vi "Power Source Settings.vi"(8 "error in":errorcluster, 10 "Action":T1(ring), 11 "COM":refnum<visa-resource-name>="COM3") -> (0 "error out":errorcluster, 3 "read buffer":string)   [LabVIEW 2014]
uses:
  <vilib>/Instr/_visa.llb/VISA Configure Serial Port (Instr).vi
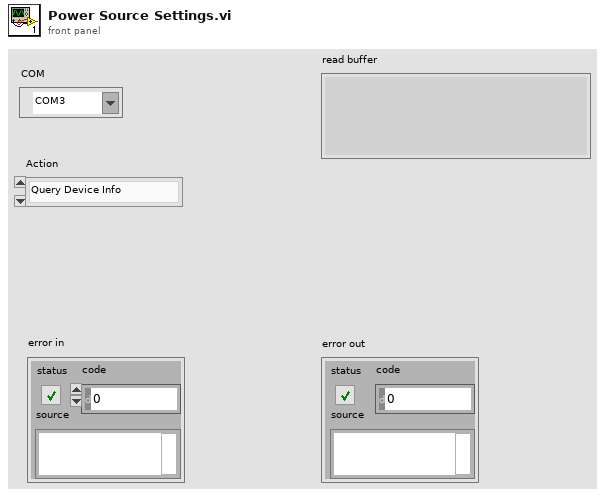
[diagram p1: front panel]
types:
  T1 = enum16{"Query Device Info", "Set Voltage", "Read Voltage", "Set Current", "Read Current", "Enable Output", "Disable Output", "Set to Remote", "Set to Local", "Get Errors", "Set Protect Voltage", "Read Protect Voltage"}
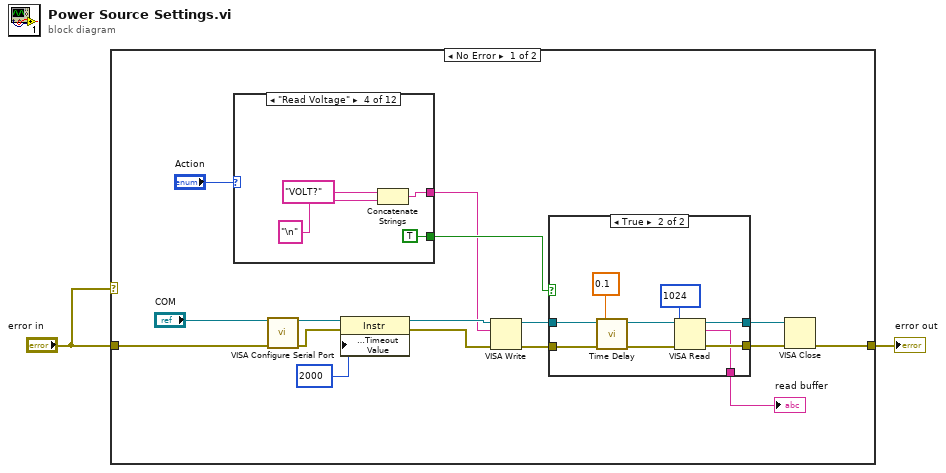
[diagram p0: block diagram]
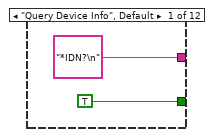
[diagram p2: hidden frame]
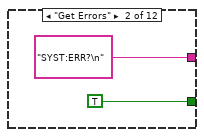
[diagram p3: hidden frame]
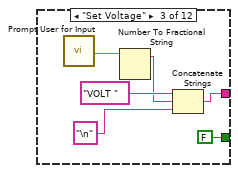
[diagram p4: hidden frame]
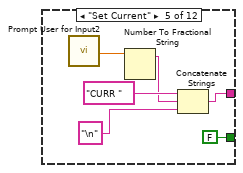
[diagram p5: hidden frame]
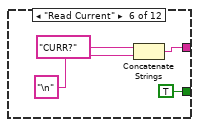
[diagram p6: hidden frame]
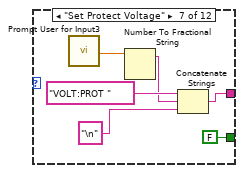
[diagram p7: hidden frame]
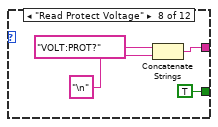
[diagram p8: hidden frame]
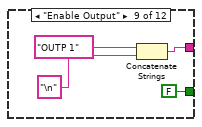
[diagram p9: hidden frame]
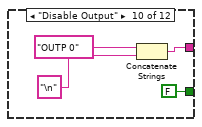
[diagram p10: hidden frame]
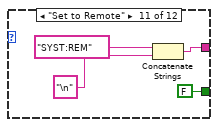
[diagram p11: hidden frame]
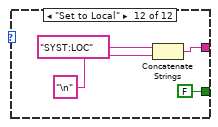
[diagram p12: hidden frame]
diagram:
  n1 = case shown="No Error" "error in" {
    tunnel: [w10 w79] -> w2
    tunnel: "error in" -> [w6 w79]
    frame No Error {
      n2 = case shown="\"Read Voltage\"" "Action" {
        tunnel: [TRUE TRUE FALSE TRUE FALSE TRUE FALSE TRUE FALSE FALSE FALSE FALSE] -> w4
        tunnel: ["*IDN?\n" ("Command") "SYST:ERR?\n" ("Command") w24 w30 w34 w40 w44 w50 w54 w58 w62 w66] -> w3
        frame "Query Device Info", Default {
        }
        frame "Get Errors" {
        }
        frame "Set Voltage" {
          n3 = call "Prompt User for Input"() -> ("电压（V)"=w27:dbl)  [unwired: 17 in, 2 out]
          n4 = Number To Fractional String(number=w27) -> (F-format string=w26:string)  [unwired: 3 in]
          n5 = Concatenate Strings("VOLT " ("Command"), w26, "\n") -> (w24:string)
        }
        frame "Read Voltage" {
          n6 = Concatenate Strings("VOLT?" ("Command"), "\n") -> (w30:string)
        }
        frame "Set Current" {
          n7 = call "Prompt User for Input2"() -> ("电流（A)"=w37:dbl)  [unwired: 17 in, 2 out]
          n8 = Number To Fractional String(number=w37) -> (F-format string=w36:string)  [unwired: 3 in]
          n9 = Concatenate Strings("CURR " ("Command"), w36, "\n") -> (w34:string)
        }
        frame "Read Current" {
          n10 = Concatenate Strings("CURR?" ("Command"), "\n") -> (w40:string)
        }
        frame "Set Protect Voltage" {
          n11 = call "Prompt User for Input3"() -> ("电压（V）"=w47:dbl)  [unwired: 17 in, 2 out]
          n12 = Number To Fractional String(number=w47) -> (F-format string=w46:string)  [unwired: 3 in]
          n13 = Concatenate Strings("VOLT:PROT " ("Command"), w46, "\n") -> (w44:string)
        }
        frame "Read Protect Voltage" {
          n14 = Concatenate Strings("VOLT:PROT?" ("Command"), "\n") -> (w50:string)
        }
        frame "Enable Output" {
          n15 = Concatenate Strings("OUTP 1" ("Command"), "\n") -> (w54:string)
        }
        frame "Disable Output" {
          n16 = Concatenate Strings("OUTP 0" ("Command"), "\n") -> (w58:string)
        }
        frame "Set to Remote" {
          n17 = Concatenate Strings("SYST:REM" ("Command"), "\n") -> (w62:string)
        }
        frame "Set to Local" {
          n18 = Concatenate Strings("SYST:LOC" ("Command"), "\n") -> (w66:string)
        }
      }
      n19 = call-poly "VISA Configure Serial Port"("VISA resource name"="COM", "error in (no error)"=w6) -> ("VISA resource name out"=w12:refnum<visa-resource-name>, "error out"=w8:errorcluster)  [unwired: 12 in]
      n20 = property class="Instr"(reference=w12, error in=w8, "General Settings:Timeout Value"=u32 2000) -> (reference out=w11:refnum<visa-resource-name>, error out=w9:errorcluster)
      n21 = VISA Write(VISA resource name=w11, write buffer=w3, error in (no error)=w9) -> (VISA resource name out=w7:refnum<visa-resource-name>, error out=w18:errorcluster)  [unwired: 1 out]
      n22 = case shown="True" w4 {
        tunnel: w18 -> [w69 w78]
        tunnel: [w69 w77] -> w17
        tunnel: [w70 w76] -> w16
        tunnel: [_ w75] -> w15
        tunnel: w7 -> [w70 w71]
        frame False {
        }
        frame True {
          n23 = call "Time Delay"("error in (no error)"=w78, "Delay Time (s)"=0.1) -> ("error out"=w73:errorcluster)  [unwired: 9 in]
          n24 = VISA Read(VISA resource name=w71, byte count=u32 1024, error in (no error)=w73) -> (VISA resource name out=w76:refnum<visa-resource-name>, read buffer=w75:string, error out=w77:errorcluster)  [unwired: 1 out]
        }
      }
      "read buffer" <- w15
      n25 = VISA Close(VISA resource name=w16, error in (no error)=w17) -> (error out=w10:errorcluster)
    }
    frame Error {
    }
  }
  "error out" <- w2
